vi "FTW-Test-JSON-ElementSet.vi"() -> ()   [LabVIEW 2015]
panel:
  out "Initialized Response String":string
  in  "Initialized Response":string
  in  "error in":errorcluster
  out "error out":errorcluster
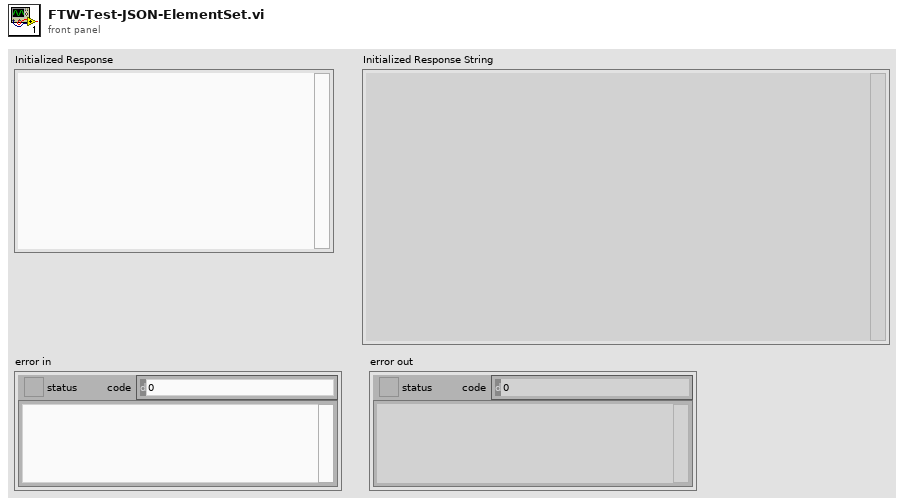
[diagram p1: front panel]
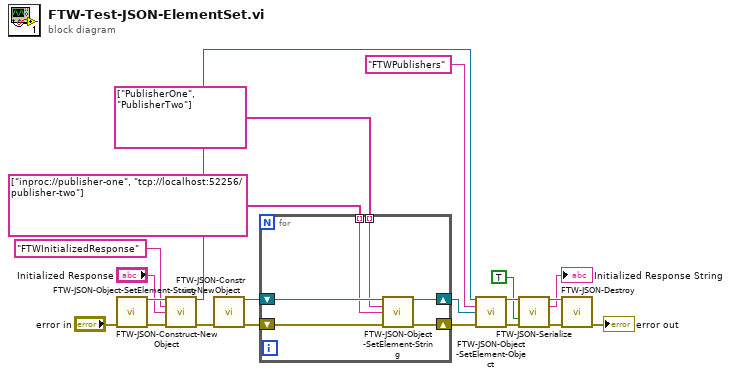
[diagram p0: block diagram]
diagram:
  n1 = call "FTW-JSON-Construct-NewObject.vi"("error in"="error in") -> ("JSON"=w19:refnum<class "FTW-Container.lvclass">, "error out"=w20:errorcluster)  [unwired: 13 in]
  n2 = call "FTW-JSON-Object-SetElement-String.vi"("JSON"=w19, "Key"="FTWInitializedResponse", "Value"="Initialized Response", "error in"=w20) -> ("JSON out"=w11:refnum<class "FTW-Container.lvclass">, "error out"=w7:errorcluster)  [unwired: 10 in]
  n3 = call "FTW-JSON-Construct-NewObject.vi"("error in"=w7) -> ("JSON"=w9:refnum<class "FTW-Container.lvclass">, "error out"=w10:errorcluster)  [unwired: 13 in]
  n4 = for {
    shift-right: [w27] -> w6
    shift-left: w10 -> [w26]
    shift-right: [w24] -> w8
    shift-left: w9 -> [w25]
    tunnel: string[] ["PublisherOne", "PublisherTwo"] -> [w23] mode=indexing
    tunnel: string[] ["inproc://publisher-one", "tcp://localhost:52256/publisher-two"] -> [w22] mode=indexing
    n5 = call "FTW-JSON-Object-SetElement-String.vi"("JSON"=w25, "Key"=w23, "Value"=w22, "error in"=w26) -> ("JSON out"=w24:refnum<class "FTW-Container.lvclass">, "error out"=w27:errorcluster)  [unwired: 10 in]
  }
  n6 = call "FTW-JSON-Object-SetElement-Object.vi"("JSON Object"=w11, "Key"="FTWPublishers", "JSON Sub-Object"=w8, "error in"=w6) -> ("JSON Root Object"=w14:refnum<class "FTW-Container.lvclass">, "error out"=w5:errorcluster)  [unwired: 10 in]
  n7 = call "FTW-JSON-Serialize.vi"("JSON"=w14, "Pretty Print"=TRUE, "error in"=w5) -> ("JSON out"=w13:refnum<class "FTW-Container.lvclass">, "JSON String (UTF-8)"=→"Initialized Response String":string, "error out"=w15:errorcluster)  [unwired: 10 in]
  n8 = call "FTW-JSON-Destroy.vi"("JSON"=w13, "error in"=w15) -> ("error out"=→"error out":errorcluster)  [unwired: 13 in]
